vi "Teleop.vi"(10 "Match Info":T1={"Autonomous Elapsed Seconds"=0.0, "TeleOp Elapsed Seconds"=0.0, "Disabled Elapsed Seconds"=0.0, "Visited Autonomous"=FALSE, "Visited TeleOp"=FALSE, "Visited Disabled"=FALSE, "Autonomous Settings"={"Autonomous Style"=enum."Independent", "VI Refnum"=refnum}}, 11 "Call Context":T2) -> ()   [LabVIEW 2012]
doc: "This VI is called for each TeleOp packet received from the DS where the robot is not disabled. It is often used to read from the joysticks and update I/O or to update setpoints for timed control loops. It should complete and return within 20 milliseconds or it may miss DS packets."
uses:
  <vilib>/Rock Robotics/WPI/DriverStation/WPI_DriverStationDerivedRobotMode.ctl
  <vilib>/Rock Robotics/WPI/DriverStation/WPI_DriverStationMatch Info.ctl
  <vilib>/Rock Robotics/WPI/Relay/WPI_RelayValue.ctl
  Robot Global Data.vi
  <vilib>/Rock Robotics/WPI/Joystick/WPI_JoystickGetSetRefNum.vi
panel:
  in  "PTO Disabled":dbl=90.0
  in  "PTO Enabled":dbl=140.0
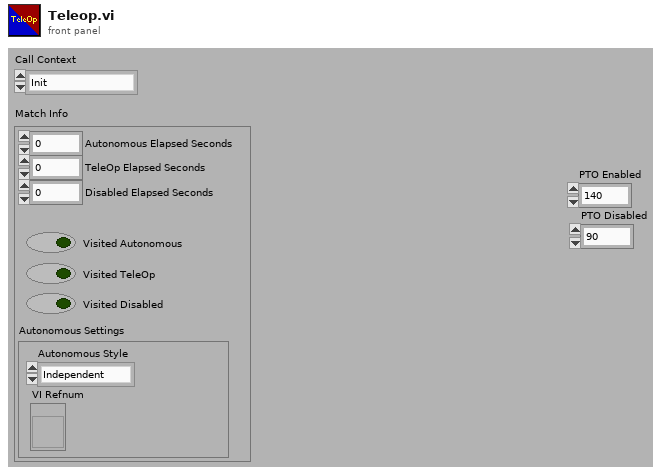
[diagram p1: front panel]
types:
  T1 = typedef "WPI_DriverStationMatch Info.ctl" = cluster{"Autonomous Elapsed Seconds":dbl, "TeleOp Elapsed Seconds":dbl, "Disabled Elapsed Seconds":dbl, "Visited Autonomous":bool, "Visited TeleOp":bool, "Visited Disabled":bool, "Autonomous Settings":cluster{"Autonomous Style":enum16{"Iterative", "Independent"}, "VI Refnum":refnum<vi>}}
  T2 = typedef "WPI_DriverStationDerivedRobotMode.ctl" = enum16{"Init", "Execute", "Stop"}
  T3 = typedef "WPI_RelayValue.ctl" = enum16{"Off", "On", "Forward", "Reverse"}
  T4 = typedef "WPI_MotorControlDeviceRef.ctl" = cluster{"DeviceStatus":errorcluster, "Type":enum16{"PWM", "CAN"}, "PWM":cluster{"Digital Module":T5, "PWM Channel":T6, "DeadBand":T7}, "CAN":cluster{"Device Number":u8, "Control Mode":T8, "Semaphore":T9, "Max Vout":dbl}, "Invert":bool, "TransformRef":T10, "InvTransformRef":T10}
  T5 = typedef "FPGA_TypedefDigitalModule.ctl" = enum16{"Digital Module 1", "Digital Module 2"}
  T6 = typedef "FPGA_DIOPWMChannel.ctl" = enum8{"PWM 1", "PWM 2", "PWM 3", "PWM 4", "PWM 5", "PWM 6", "PWM 7", "PWM 8", "PWM 9", "PWM 10", "Invalid"}
  T7 = typedef "WPI_PWMDeadband.ctl" = cluster{"Name":string, "maxPositivePwm":i32, "minPositivePwm":i32, "centerPwm":i32, "maxNegativePwm":i32, "minNegativePwm":i32, "angularRange":u16}
  T8 = typedef "WPI_CANJaguar_ControlMode.ctl" = enum8{"Percent VBus", "Current", "Speed", "Position", "Voltage"}
  T9 = typedef "Semaphore RefNum" = refnum<k1>
  T10 = typedef "WPI_PWMTransform_ConPane.ctl" = refnum<vi>
  T11 = typedef "WPI_RelayDevRef.ctl" = cluster{"DevStatus":errorcluster, "Relay Channel":T12, "Digital Module":T5, "Relay Direction":T13}
  T12 = typedef "FPGA_DIORelayChannel.ctl" = enum8{"Relay 1", "Relay 2", "Relay 3", "Relay 4", "Relay 5", "Relay 6", "Relay 7", "Relay 8", "Invalid"}
  T13 = typedef "WPI_RelayDirection.ctl" = enum16{"Both directions", "Forward only", "Reverse only"}
  T14 = cluster{"Driver Station Digital Input (1-8)[0]":bool, "Driver Station Digital Input (1-8)[1]":bool, "Driver Station Digital Input (1-8)[2]":bool, "Driver Station Digital Input (1-8)[3]":bool, "Driver Station Digital Input (1-8)[4]":bool, "Driver Station Digital Input (1-8)[5]":bool, "Driver Station Digital Input (1-8)[6]":bool, "Driver Station Digital Input (1-8)[7]":bool, "Driver Station Digital Input (1-8)[8]":bool}
  T15 = typedef "WPI_JoystickDevRef.ctl" = cluster{"Device":T16}
  T16 = typedef "WPI_JoystickDeviceEnum.ctl" = enum16{"USB 1", "USB 2", "USB 3", "USB 4", "Kinect 1", "Kinect 2"}
  T17 = cluster{"axis 1 (x)":dbl, "axis 2 (y)":dbl, "axis 3 (throttle)":dbl, "axis 4":dbl, "axis 5":dbl, "axis 6":dbl}
  T18 = typedef "WPI_JoystickButtonState.ctl" = cluster{"Button 1":bool, "Button 2":bool, "Button 3":bool, "Button 4":bool, "Button 5":bool, "Button 6":bool, "Button 7":bool, "Button 8":bool, "Button 9":bool, "Button 10":bool, "Button 11":bool, "Button 12":bool}
  T19 = typedef "WPI_ServoDeviceRef.ctl" = cluster{"DeviceStatus":errorcluster, "Digital Module":T5, "PWM Channel":T6, "DeadBand":T7}
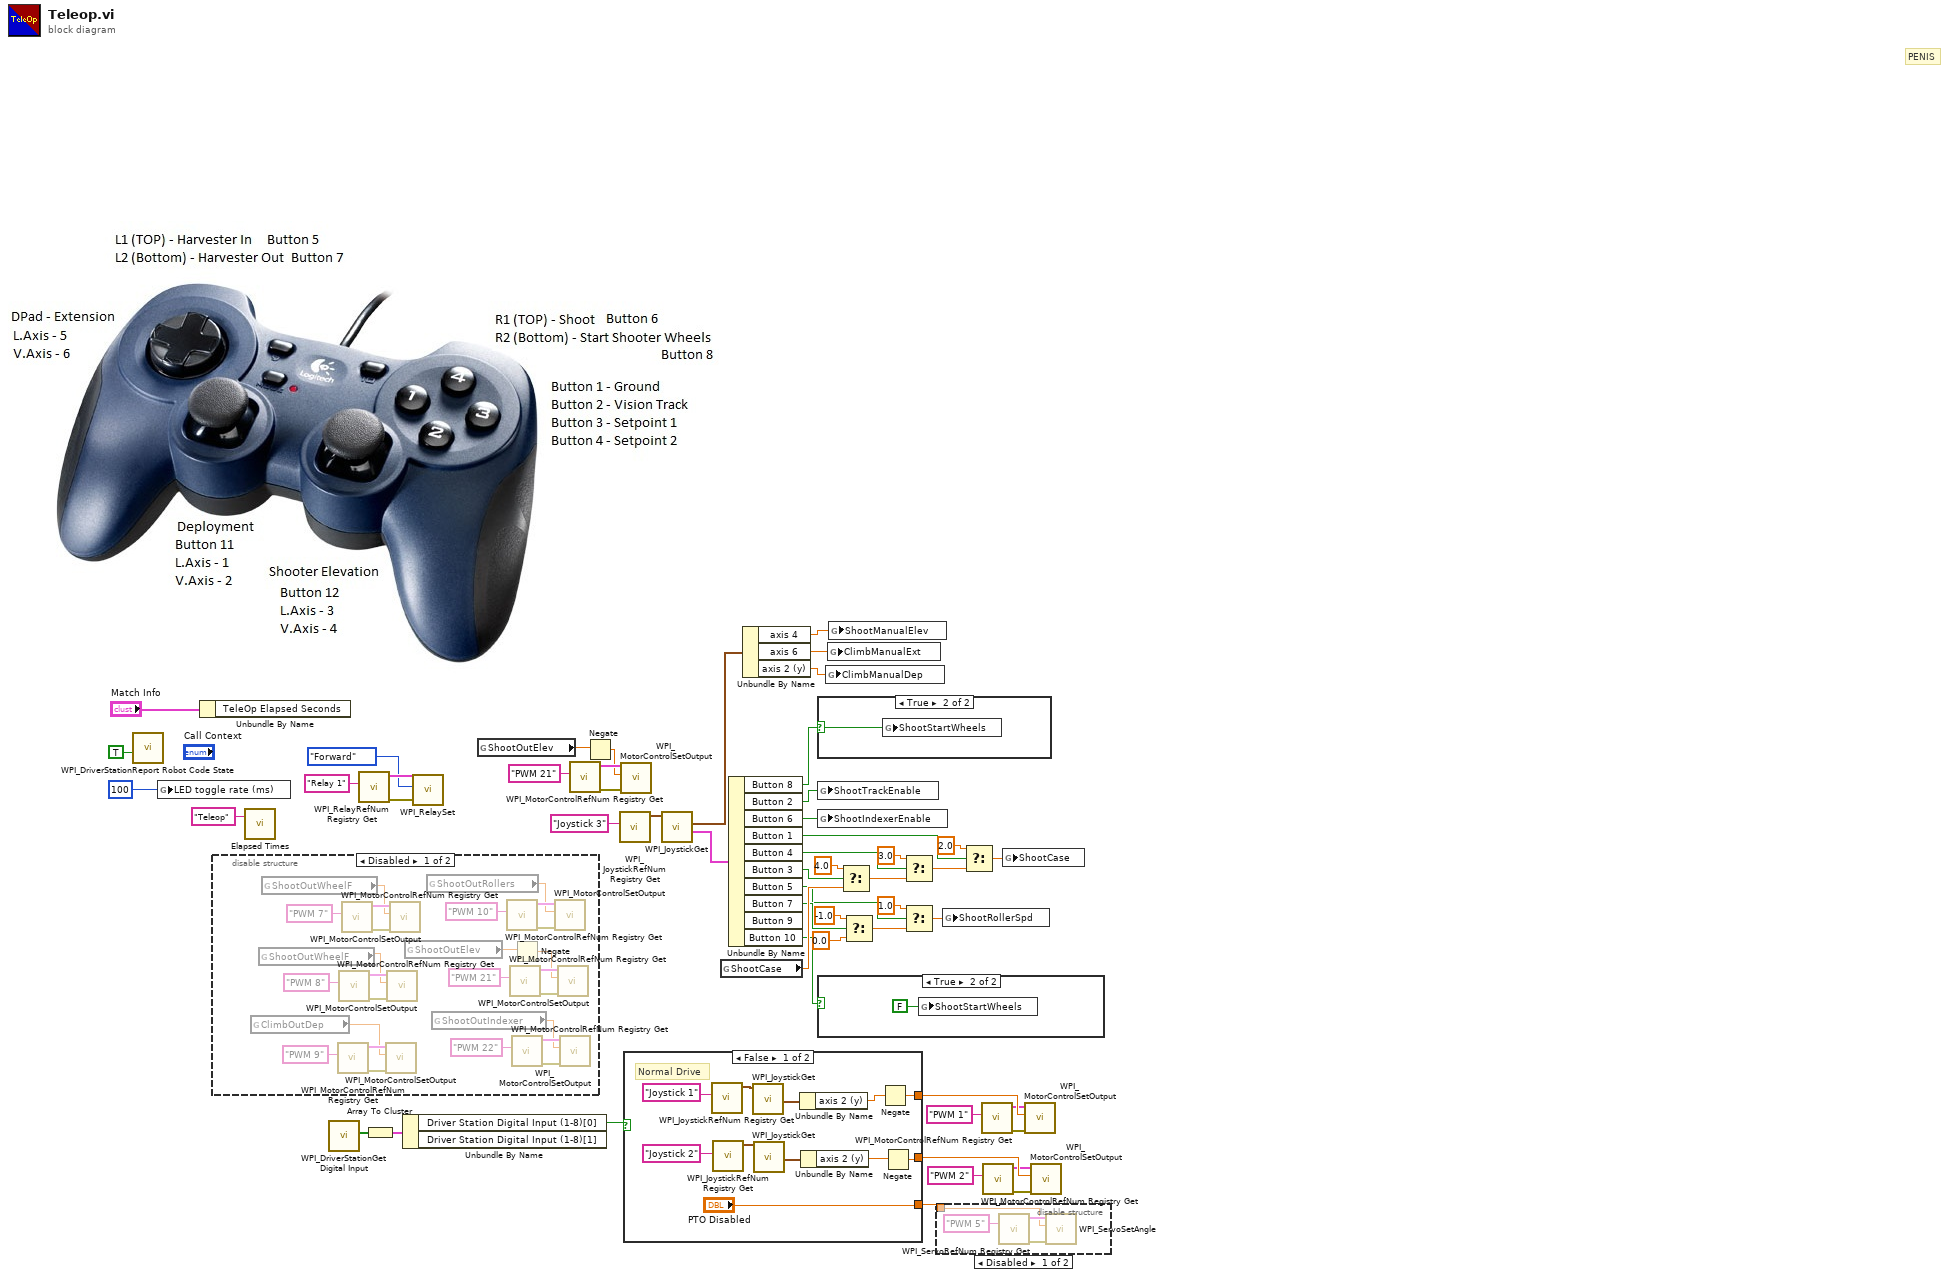
[diagram p0: block diagram]
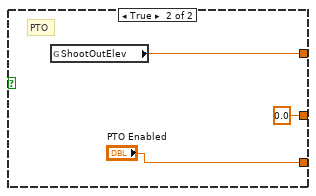
[diagram p3: hidden frame]
diagram:
  # "PENIS"
  n1 = call <vilib>:"WPI_DriverStationReport Robot Code State.vi"("TeleOp"=TRUE ("Autonomous")) -> ()  [unwired: 10 in, 1 out]
  n2 = global write "Robot Global Data.vi" "LED toggle rate (ms)"(u32 100 ("LED ms toggle rate")) -> ()
  n3 = Unbundle By Name("Match Info") -> ()  [unwired: 1 out]
  n4 = disable-structure shown="Disabled" {
    frame Disabled {
      n5 = global read "Robot Global Data.vi" "ClimbOutDep"() -> (w54:dbl)
      n6 = global read "Robot Global Data.vi" "ShootOutWheelF"() -> (w55:dbl)
      n7 = global read "Robot Global Data.vi" "ShootOutWheelF"() -> (w60:dbl)
      n8 = call <vilib>:"WPI_MotorControlRefNum Registry Get.vi"("refnum name"="PWM 9") -> ("error out"=w72:errorcluster, "MotorControlDevRef"=w71:T4)  [unwired: 9 in]
      n9 = call <vilib>:"WPI_MotorControlRefNum Registry Get.vi"("refnum name"="PWM 8") -> ("error out"=w73:errorcluster, "MotorControlDevRef"=w74:T4)  [unwired: 9 in]
      n10 = call <vilib>:"WPI_MotorControlRefNum Registry Get.vi"("refnum name"="PWM 7") -> ("error out"=w78:errorcluster, "MotorControlDevRef"=w77:T4)  [unwired: 9 in]
      n11 = call <vilib>:"WPI_MotorControlSetOutput.vi"("error in (no error)"=w72, "Output"=w54, "MotorControlDevRef"=w71) -> ()  [unwired: 6 in, 3 out]
      n12 = call <vilib>:"WPI_MotorControlSetOutput.vi"("error in (no error)"=w73, "Output"=w55, "MotorControlDevRef"=w74) -> ()  [unwired: 6 in, 3 out]
      n13 = call <vilib>:"WPI_MotorControlSetOutput.vi"("error in (no error)"=w78, "Output"=w60, "MotorControlDevRef"=w77) -> ()  [unwired: 6 in, 3 out]
      n14 = global read "Robot Global Data.vi" "ShootOutElev"() -> (w57:dbl)
      n15 = global read "Robot Global Data.vi" "ShootOutRollers"() -> (w58:dbl)
      n16 = global read "Robot Global Data.vi" "ShootOutIndexer"() -> (w59:dbl)
      n17 = call <vilib>:"WPI_MotorControlRefNum Registry Get.vi"("refnum name"="PWM 10") -> ("error out"=w67:errorcluster, "MotorControlDevRef"=w68:T4)  [unwired: 9 in]
      n18 = call <vilib>:"WPI_MotorControlRefNum Registry Get.vi"("refnum name"="PWM 21") -> ("error out"=w66:errorcluster, "MotorControlDevRef"=w65:T4)  [unwired: 9 in]
      n19 = Negate(x=w57) -> (-x=w56:dbl)
      n20 = call <vilib>:"WPI_MotorControlRefNum Registry Get.vi"("refnum name"="PWM 22") -> ("error out"=w61:errorcluster, "MotorControlDevRef"=w62:T4)  [unwired: 9 in]
      n21 = call <vilib>:"WPI_MotorControlSetOutput.vi"("error in (no error)"=w67, "Output"=w58, "MotorControlDevRef"=w68) -> ()  [unwired: 6 in, 3 out]
      n22 = call <vilib>:"WPI_MotorControlSetOutput.vi"("error in (no error)"=w66, "Output"=w56, "MotorControlDevRef"=w65) -> ()  [unwired: 6 in, 3 out]
      n23 = call <vilib>:"WPI_MotorControlSetOutput.vi"("error in (no error)"=w61, "Output"=w59, "MotorControlDevRef"=w62) -> ()  [unwired: 6 in, 3 out]
    }
    frame Enabled {
    }
  }
  n24 = call "Elapsed Times.vi"("Call Name"="Teleop") -> ()  [unwired: 2 in, 1 out]
  n25 = call <vilib>:"WPI_DriverStationGet Digital Input.vi"() -> ("Driver Station Digital Input (1-8)"=w13:bool[])  [unwired: 11 in]
  n26 = call <vilib>:"WPI_RelayRefNum Registry Get.vi"("refnum name"="Relay 1") -> ("error out"=w48:errorcluster, "RelayDevRef"=w50:T11)  [unwired: 9 in]
  n27 = Array To Cluster(array=w13) -> (cluster=w12:T14)
  n28 = Unbundle By Name(w12) -> ("Driver Station Digital Input (1-8)[0]"=w11:bool)  [unwired: 1 out]
  n29 = call <vilib>:"WPI_RelaySet.vi"("error in (no error)"=w48, "RelayValue"=WPI_RelayValue."Forward", "RelayDevRef"=w50) -> ()  [unwired: 7 in, 2 out]
  n30 = global read "Robot Global Data.vi" "ShootOutElev"() -> (w25:dbl)
  n31 = call <vilib>:"WPI_MotorControlRefNum Registry Get.vi"("refnum name"="PWM 21") -> ("error out"=w28:errorcluster, "MotorControlDevRef"=w27:T4)  [unwired: 9 in]
  n32 = Negate(x=w25) -> (-x=w24:dbl)
  n33 = call <vilib>:"WPI_JoystickRefNum Registry Get.vi"("refnum name"="Joystick 3") -> ("JoystickDevRef"=w46:T15)  [unwired: 9 in, 1 out]
  n34 = call <vilib>:"WPI_MotorControlSetOutput.vi"("error in (no error)"=w28, "Output"=w24, "MotorControlDevRef"=w27) -> ()  [unwired: 6 in, 3 out]
  n35 = case shown="False" w11 {
    tunnel: [w81 w91] -> w8
    tunnel: [w80 0.0] -> w5
    tunnel: ["PTO Disabled" "PTO Enabled"] -> w2
    frame False {
      # "Normal Drive"
      n36 = call <vilib>:"WPI_JoystickRefNum Registry Get.vi"("refnum name"="Joystick 1") -> ("JoystickDevRef"=w83:T15)  [unwired: 1 in, 9 out]
      n37 = call <vilib>:"WPI_JoystickRefNum Registry Get.vi"("refnum name"="Joystick 2") -> ("JoystickDevRef"=w86:T15)  [unwired: 1 in, 9 out]
      n38 = call <vilib>:"WPI_JoystickGet.vi"("JoystickDevRef"=w83) -> ("Axes"=w84:T17)  [unwired: 1 in, 5 out]
      n39 = call <vilib>:"WPI_JoystickGet.vi"("JoystickDevRef"=w86) -> ("Axes"=w85:T17)  [unwired: 1 in, 5 out]
      n40 = Unbundle By Name(w84) -> ("axis 2 (y)"=w89:dbl)
      n41 = Unbundle By Name(w85) -> ("axis 2 (y)"=w88:dbl)
      n42 = Negate(x=w89) -> (-x=w81:dbl)
      n43 = Negate(x=w88) -> (-x=w80:dbl)
    }
    frame True {
      # "PTO"
      n44 = global read "Robot Global Data.vi" "ShootOutElev"() -> (w91:dbl)
    }
  }
  n45 = call <vilib>:"WPI_JoystickGet.vi"("JoystickDevRef"=w46) -> ("Buttons"=w44:T18, "Axes"=w43:T17)  [unwired: 4 in, 1 out]
  n46 = global read "Robot Global Data.vi" "ShootCase"() -> (w30:dbl)
  n47 = Unbundle By Name(w44) -> ("Button 8"=w15:bool, "Button 2"=w41:bool, "Button 6"=w42:bool, "Button 1"=w38:bool, "Button 4"=w36:bool, "Button 3"=w35:bool, "Button 5"=w20:bool, "Button 7"=w22:bool, "Button 10"=w14:bool)  [unwired: 1 out]
  n48 = Unbundle By Name(w43) -> ("axis 4"=w40:dbl, "axis 6"=w39:dbl, "axis 2 (y)"=w1:dbl)
  n49 = case shown="True" w15 {
    selector: w15 -> [_ w93]
    frame False {
    }
    frame True {
      n50 = global write "Robot Global Data.vi" "ShootStartWheels"(w93) -> ()
    }
  }
  n51 = global write "Robot Global Data.vi" "ShootTrackEnable"(w41) -> ()
  n52 = global write "Robot Global Data.vi" "ShootIndexerEnable"(w42) -> ()
  n53 = case shown="True" w14 {
    frame False {
    }
    frame True {
      n54 = global write "Robot Global Data.vi" "ShootStartWheels"(FALSE ("ShootStartWheels")) -> ()
    }
  }
  n55 = global write "Robot Global Data.vi" "ClimbManualDep"(w1) -> ()
  n56 = global write "Robot Global Data.vi" "ClimbManualExt"(w39) -> ()
  n57 = global write "Robot Global Data.vi" "ShootManualElev"(w40) -> ()
  n58 = Select(t=4.0, s=w35, f=w30) -> (s? t:f=w34:dbl)
  n59 = Select(t=-1.0, s=w22, f=0.0) -> (s? t:f=w21:dbl)
  n60 = Select(t=3.0, s=w36, f=w34) -> (s? t:f=w32:dbl)
  n61 = Select(t=1.0, s=w20, f=w21) -> (s? t:f=w16:dbl)
  n62 = disable-structure shown="Disabled" {
    disable-tunnel: w2 -> [w96 _]
    frame Disabled {
      n63 = call <vilib>:"WPI_ServoRefNum Registry Get.vi"("refnum name"="PWM 5") -> ("error out"=w98:errorcluster, "ServoDeviceRef"=w97:T19)  [unwired: 9 in]
      n64 = call <vilib>:"WPI_ServoSetAngle.vi"("error in (no error)"=w98, "Angle"=w96, "ServoDeviceRef"=w97) -> ()  [unwired: 7 in, 2 out]
    }
    frame Enabled {
    }
  }
  n65 = global write "Robot Global Data.vi" "ShootRollerSpd"(w16) -> ()
  n66 = Select(t=2.0, s=w38, f=w32) -> (s? t:f=w29:dbl)
  n67 = call <vilib>:"WPI_MotorControlRefNum Registry Get.vi"("refnum name"="PWM 1") -> ("error out"=w6:errorcluster, "MotorControlDevRef"=w7:T4)  [unwired: 9 in]
  n68 = call <vilib>:"WPI_MotorControlRefNum Registry Get.vi"("refnum name"="PWM 2") -> ("error out"=w3:errorcluster, "MotorControlDevRef"=w4:T4)  [unwired: 9 in]
  n69 = global write "Robot Global Data.vi" "ShootCase"(w29) -> ()
  n70 = call <vilib>:"WPI_MotorControlSetOutput.vi"("error in (no error)"=w6, "Output"=w8, "MotorControlDevRef"=w7) -> ()  [unwired: 6 in, 3 out]
  n71 = call <vilib>:"WPI_MotorControlSetOutput.vi"("error in (no error)"=w3, "Output"=w5, "MotorControlDevRef"=w4) -> ()  [unwired: 6 in, 3 out]
